vi "Pix2U32.vi"(10 "error in (no error)":errorcluster, 11 "input cluster":T1) -> (2 "error out":errorcluster, 3 "appended array":u32[](array[numeric]))   [LabVIEW 2019]
uses:
  <vilib>/picture/picture.llb/imagedata.ctl
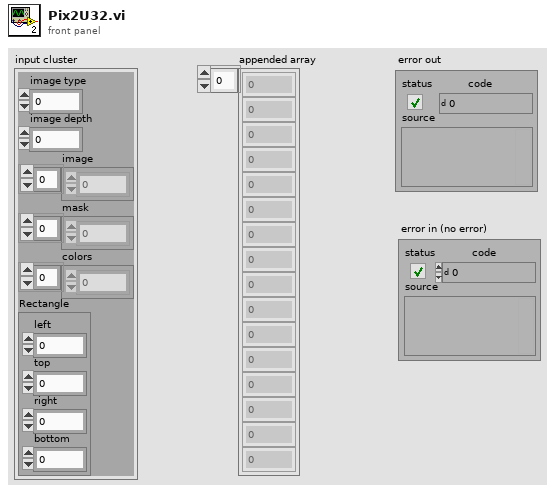
[diagram p1: front panel]
types:
  T1 = typedef "imagedata.ctl" = cluster{"image type":i32, "image depth":i32, "image":u8[], "mask":u8[], "colors":u32[], "Rectangle":cluster{"left":i16, "top":i16, "right":i16, "bottom":i16}}
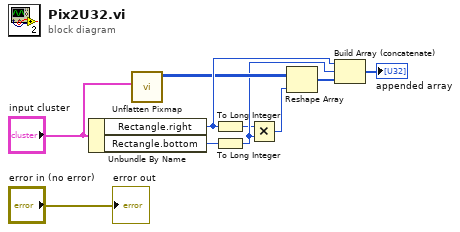
[diagram p0: block diagram]
diagram:
  n1 = Unbundle By Name("input cluster") -> ("Rectangle.right"=w8:i16, "Rectangle.bottom"=w7:i16)
  n2 = call <vilib>:"Unflatten Pixmap.vi"("image data"="input cluster") -> ("24-bit pixmap"=w5:u32[][])  [unwired: 4 in, 6 out]
  n3 = To Long Integer(number=w8) -> (32bit integer=w1:i32)
  n4 = To Long Integer(number=w7) -> (32bit integer=w2:i32)
  n5 = Multiply(x=w1, y=w2) -> (x*y=w10:i32)
  n6 = Reshape Array(w5, w10) -> (w9:u32[])
  n7 = Build Array (concatenate)(w8, w2, w9) -> (→"appended array":u32[])
  "error out" <- "error in (no error)"
